vi "Stream_CheckComplete.vi"(7 "Qbus in":refnum<class "Qbus.lvclass">, 8 "error in (no error)":errorcluster, 10 "stream Id":string, 11 "streams in":variant) -> (0 "error out":errorcluster, 3 "streams out":variant)   [LabVIEW 2017, in "FileManager.lvlib"]
uses:
  <vilib>/addons/InsightCM/Devices/Shared/Common/FileManager/FileManager.lvlib
  <vilib>/addons/Qbus/Qbus.lvclass
  <vilib>/addons/InsightCM/Devices/Shared/Common/FileManager/controls/StreamState.ctl
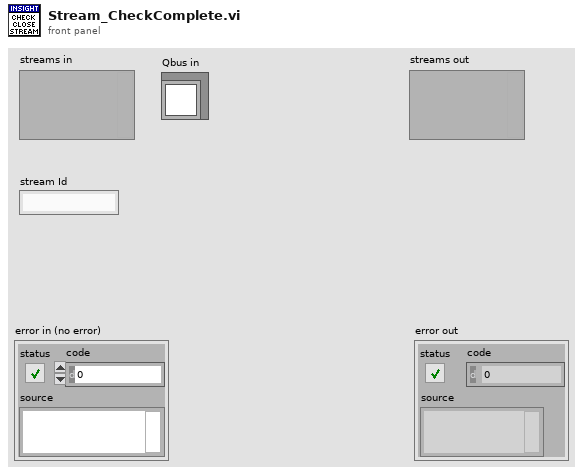
[diagram p1: front panel]
types:
  T1 = typedef "FileManager.lvlib/StreamState.ctl" = cluster{"DataGroup":string, "Stream Id":string, "LastBlock":bool, "TotalBlocks":i32, "BlocksSent":i32, "Device":string}
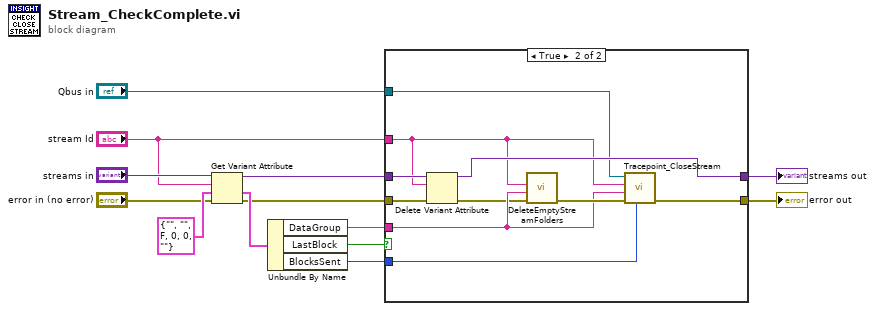
[diagram p0: block diagram]
diagram:
  n1 = Get Variant Attribute(Variant="streams in", name="stream Id", default value (empty Variant)=T1 {"DataGroup"="", "Stream Id"="", "LastBlock"=FALSE, "TotalBlocks"=0, "BlocksSent"=0, "Device"=""} ("Stream"), error in="error in (no error)") -> (duplicate Variant=w8:variant, value=w11:T1, error out=w9:errorcluster)  [unwired: 1 out]
  n2 = Unbundle By Name(w11) -> ("DataGroup"=w2:string, "LastBlock"=w1:bool, "BlocksSent"=w7:i32)
  n3 = case shown="True" w1 {
    tunnel: w9 -> [w14 w25]
    tunnel: w8 -> [w15 w24]
    tunnel: w7 -> [_ w17]
    tunnel: "Qbus in" -> [_ w19]
    tunnel: [w15 w23] -> w5
    tunnel: [w14 w18] -> w4
    tunnel: "stream Id" -> [_ w20]
    tunnel: w2 -> [_ w21]
    frame False {
    }
    frame True {
      # "Close Stream"
      n4 = Delete Variant Attribute(4:w25, 6:w20, 7:w24) -> (0:w16:errorcluster, 3:w23:variant)  [unwired: 1 out]
      n5 = call <vilib>:"DeleteEmptyStreamFolders.vi"("error in (no error)"=w16, "data group"=w21, "stream Id"=w20) -> ("error out"=w22:errorcluster)  [unwired: 8 in]
      n6 = call <vilib>:"Tracepoint_CloseStream.vi"("blocks sent"=w17, "error in (no error)"=w22, "group"=w21, "stream Id"=w20, "Qbus in"=w19) -> ("error out"=w18:errorcluster)  [unwired: 6 in]
    }
  }
  "streams out" <- w5
  "error out" <- w4
